vi "AnalogRead.vi"(3 "error in (no error)":errorcluster, 4 "Data Out Mode":enum16{"Normalized", "Voltage", "Binary"}(ring), 5 "Channel":u8=1, 6 "VISA Refnum in":refnum<visa-resource-name>) -> (0 "error out":errorcluster, 1 "Numeric":dbl, 2 "VISA Refnum out":refnum<visa-resource-name>)   [LabVIEW 2016]
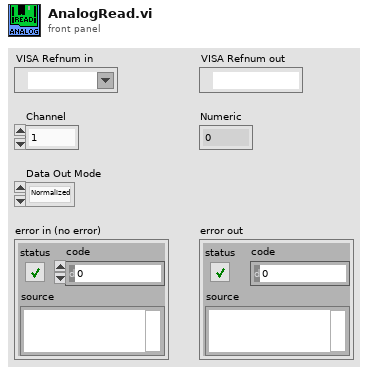
[diagram p1: front panel]
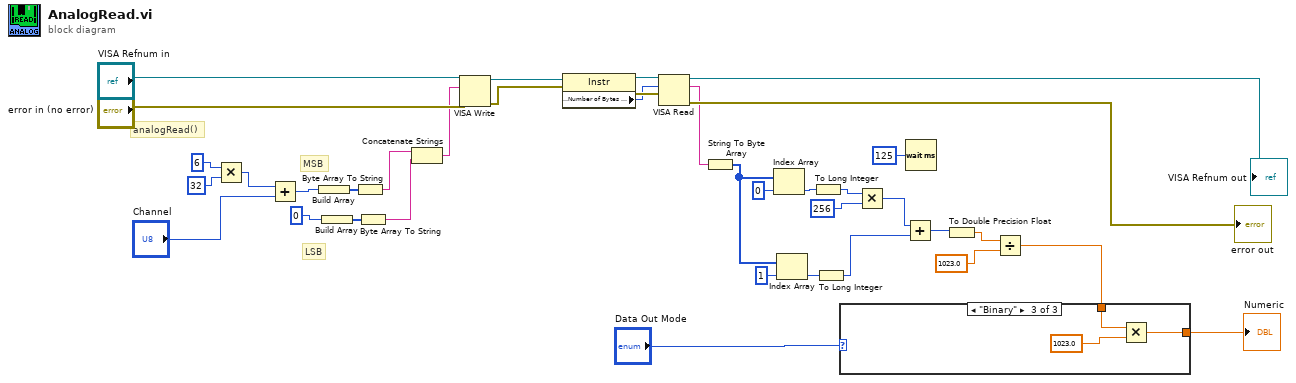
[diagram p0: block diagram]
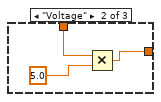
[diagram p3: hidden frame]
diagram:
  # "LSB"
  # "MSB"
  # "analogRead()"
  n1 = Multiply(x=u8 6, y=u8 32) -> (x*y=w2:u8)
  n2 = Add(x=w2, y="Channel") -> (x+y=w1:u8)
  n3 = Build Array(w1) -> (w11:u8[])
  n4 = Build Array(u8 0) -> (w15:u8[])
  n5 = Byte Array To String(unsigned byte array=w11) -> (string=w12:string)
  n6 = Byte Array To String(unsigned byte array=w15) -> (string=w16:string)
  n7 = Concatenate Strings(w12, w16) -> (w13:string)
  n8 = VISA Write(VISA resource name="VISA Refnum in", write buffer=w13, error in (no error)="error in (no error)") -> (VISA resource name out=w5:refnum<visa-resource-name>, error out=w4:errorcluster)  [unwired: 1 out]
  n9 = property class="Instr"(reference=w5, error in=w4) -> (reference out=w8:refnum<visa-resource-name>, error out=w7:errorcluster, "Serial Settings:Number of Bytes at Serial Port"=w6:u32)
  n10 = VISA Read(VISA resource name=w8, byte count=w6, error in (no error)=w7) -> (VISA resource name out=→"VISA Refnum out":refnum<visa-resource-name>, read buffer=w14:string, error out=→"error out":errorcluster)  [unwired: 1 out]
  n11 = String To Byte Array(string=w14) -> (unsigned byte array=w22:u8[])
  n12 = Index Array(array=w22, index=0) -> (element=w25:u8)
  n13 = Index Array(array=w22, index=1) -> (element=w30:u8)
  n14 = To Long Integer(number=w25) -> (32bit integer=w26:i32)
  n15 = To Long Integer(number=w30) -> (32bit integer=w29:i32)
  n16 = Multiply(x=w26, y=256) -> (x*y=w28:i32)
  n17 = Add(x=w28, y=w29) -> (x+y=w31:i32)
  n18 = Wait (ms)(milliseconds to wait=u32 125) -> ()  [unwired: 1 out]
  n19 = To Double Precision Float(number=w31) -> (double precision float=w32:dbl)
  n20 = Divide(x=w32, y=1023.0) -> (x/y=w36:dbl)
  n21 = case shown="\"Binary\"" "Data Out Mode" {
    tunnel: w36 -> [w38 w41 w44]
    tunnel: [w38 w39 w43] -> w37
    frame "Normalized", Default {
    }
    frame "Voltage" {
      n22 = Multiply(x=w41, y=5.0) -> (x*y=w39:dbl)
    }
    frame "Binary" {
      n23 = Multiply(x=w44, y=1023.0) -> (x*y=w43:dbl)
    }
  }
  "Numeric" <- w37
